vi "JSON String to Compiled Settings.vi"(7 "CompiledSettings":cluster{"Name":string}, 8 "error in":errorcluster, 11 "JSON":string) -> (0 "error out":errorcluster, 3 "CompiledSettingsOut":cluster{"Name":string})   [LabVIEW 2026, in "Template Debug Tools.lvlib"]
doc: "Convert JSON to the LabVIEW Data Type entered.\n\nStrings or Arrays of strings marked with a leading \"<JSON>\" tag in their name (including inside clusters) are returnd as JSON. \n\nStrings or Arrays of strings marked with a leading \"<UTF8>\" tag in their name (including inside clusters) are returned encoded as UTF-8 (rather than the standard LabVIEW encoding)."
uses:
  Template Debug Tools.lvlib
  <vilib>/JDP Science/JSONtext/JSONtext.lvlib
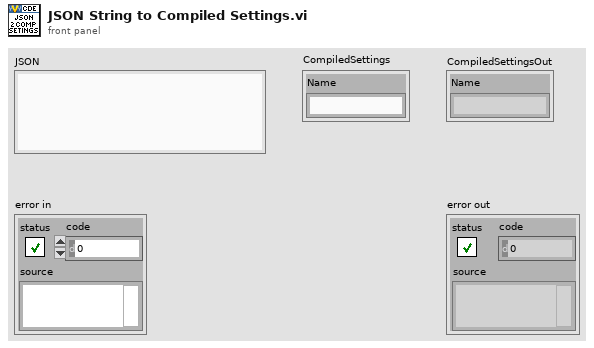
[diagram p1: front panel]
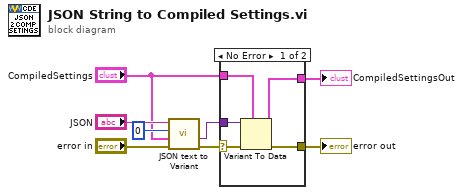
[diagram p0: block diagram]
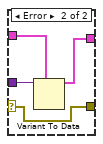
[diagram p2: hidden frame]
diagram:
  n1 = call <vilib>:"JSON text to Variant.vi"("error in (no error)"="error in", "Data Type"="CompiledSettings", "Offset"=0, "JSON"="JSON") -> ("error out"=w1:errorcluster, "Variant out"=w3:variant)  [unwired: 6 in]
  n2 = case shown="No Error" w1 {
    selector: w1 -> [w9 w14]
    tunnel: [w13 w14] -> w5
    tunnel: "CompiledSettings" -> [w12 w17]
    tunnel: w3 -> [w11 w16]
    tunnel: [w10 w15] -> w2
    frame No Error {
      n3 = Variant To Data(error in=w9, type=w12, Variant=w11) -> (data=w10:cluster{"Name":string}, error out=w13:errorcluster)
    }
    frame Error {
      n4 = Variant To Data(type=w17, Variant=w16) -> (data=w15:cluster{"Name":string})  [unwired: 1 in, 1 out]
    }
  }
  "CompiledSettingsOut" <- w2
  "error out" <- w5
